vi "display_1s_stim_9s_ISI_CS1_CS2_no_trigger_with_probes.vi"() -> ()   [LabVIEW 2019]
uses:
  <vilib>/Analysis/Matrix/Datatypes/RealMatrix.ctl
  <vilib>/Utility/file.llb/Write Delimited Spreadsheet (DBL).vi
  <vilib>/Analysis/Matrix/NI_Matrix.lvlib
panel:
  out "Num trials":u32=204
  out "ISI Time":dbl
  out "Stim TS":dbl
  out "Output":dbl[][](array[numeric])
  out "Output frame":T1
  out "Array temp1":T1
  out "Elapsed Time":dbl
  out "Display":bool=TRUE
  out "Trial":u32=1
  out "reward":dbl[](array[numeric])
  out "stim_id":dbl[](array[numeric])
  out "stim_loaded":dbl
  out "Timings":dbl[](array[numeric])
  out "Stimuli Loaded?":bool
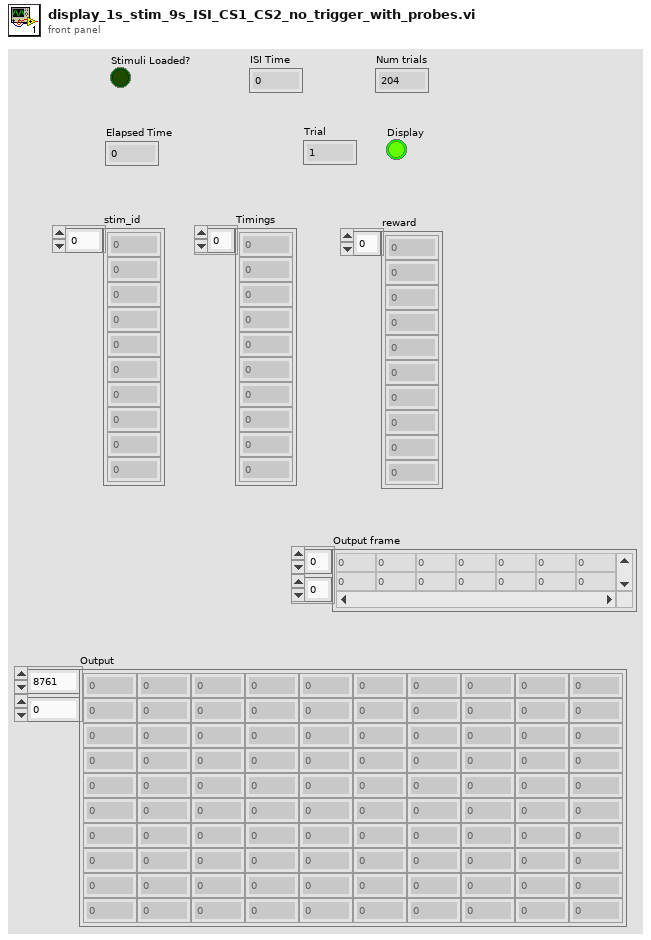
[diagram p1: front panel]
types:
  T1 = typedef "NI_Matrix.lvlib/RealMatrix.ctl" = dbl[][]
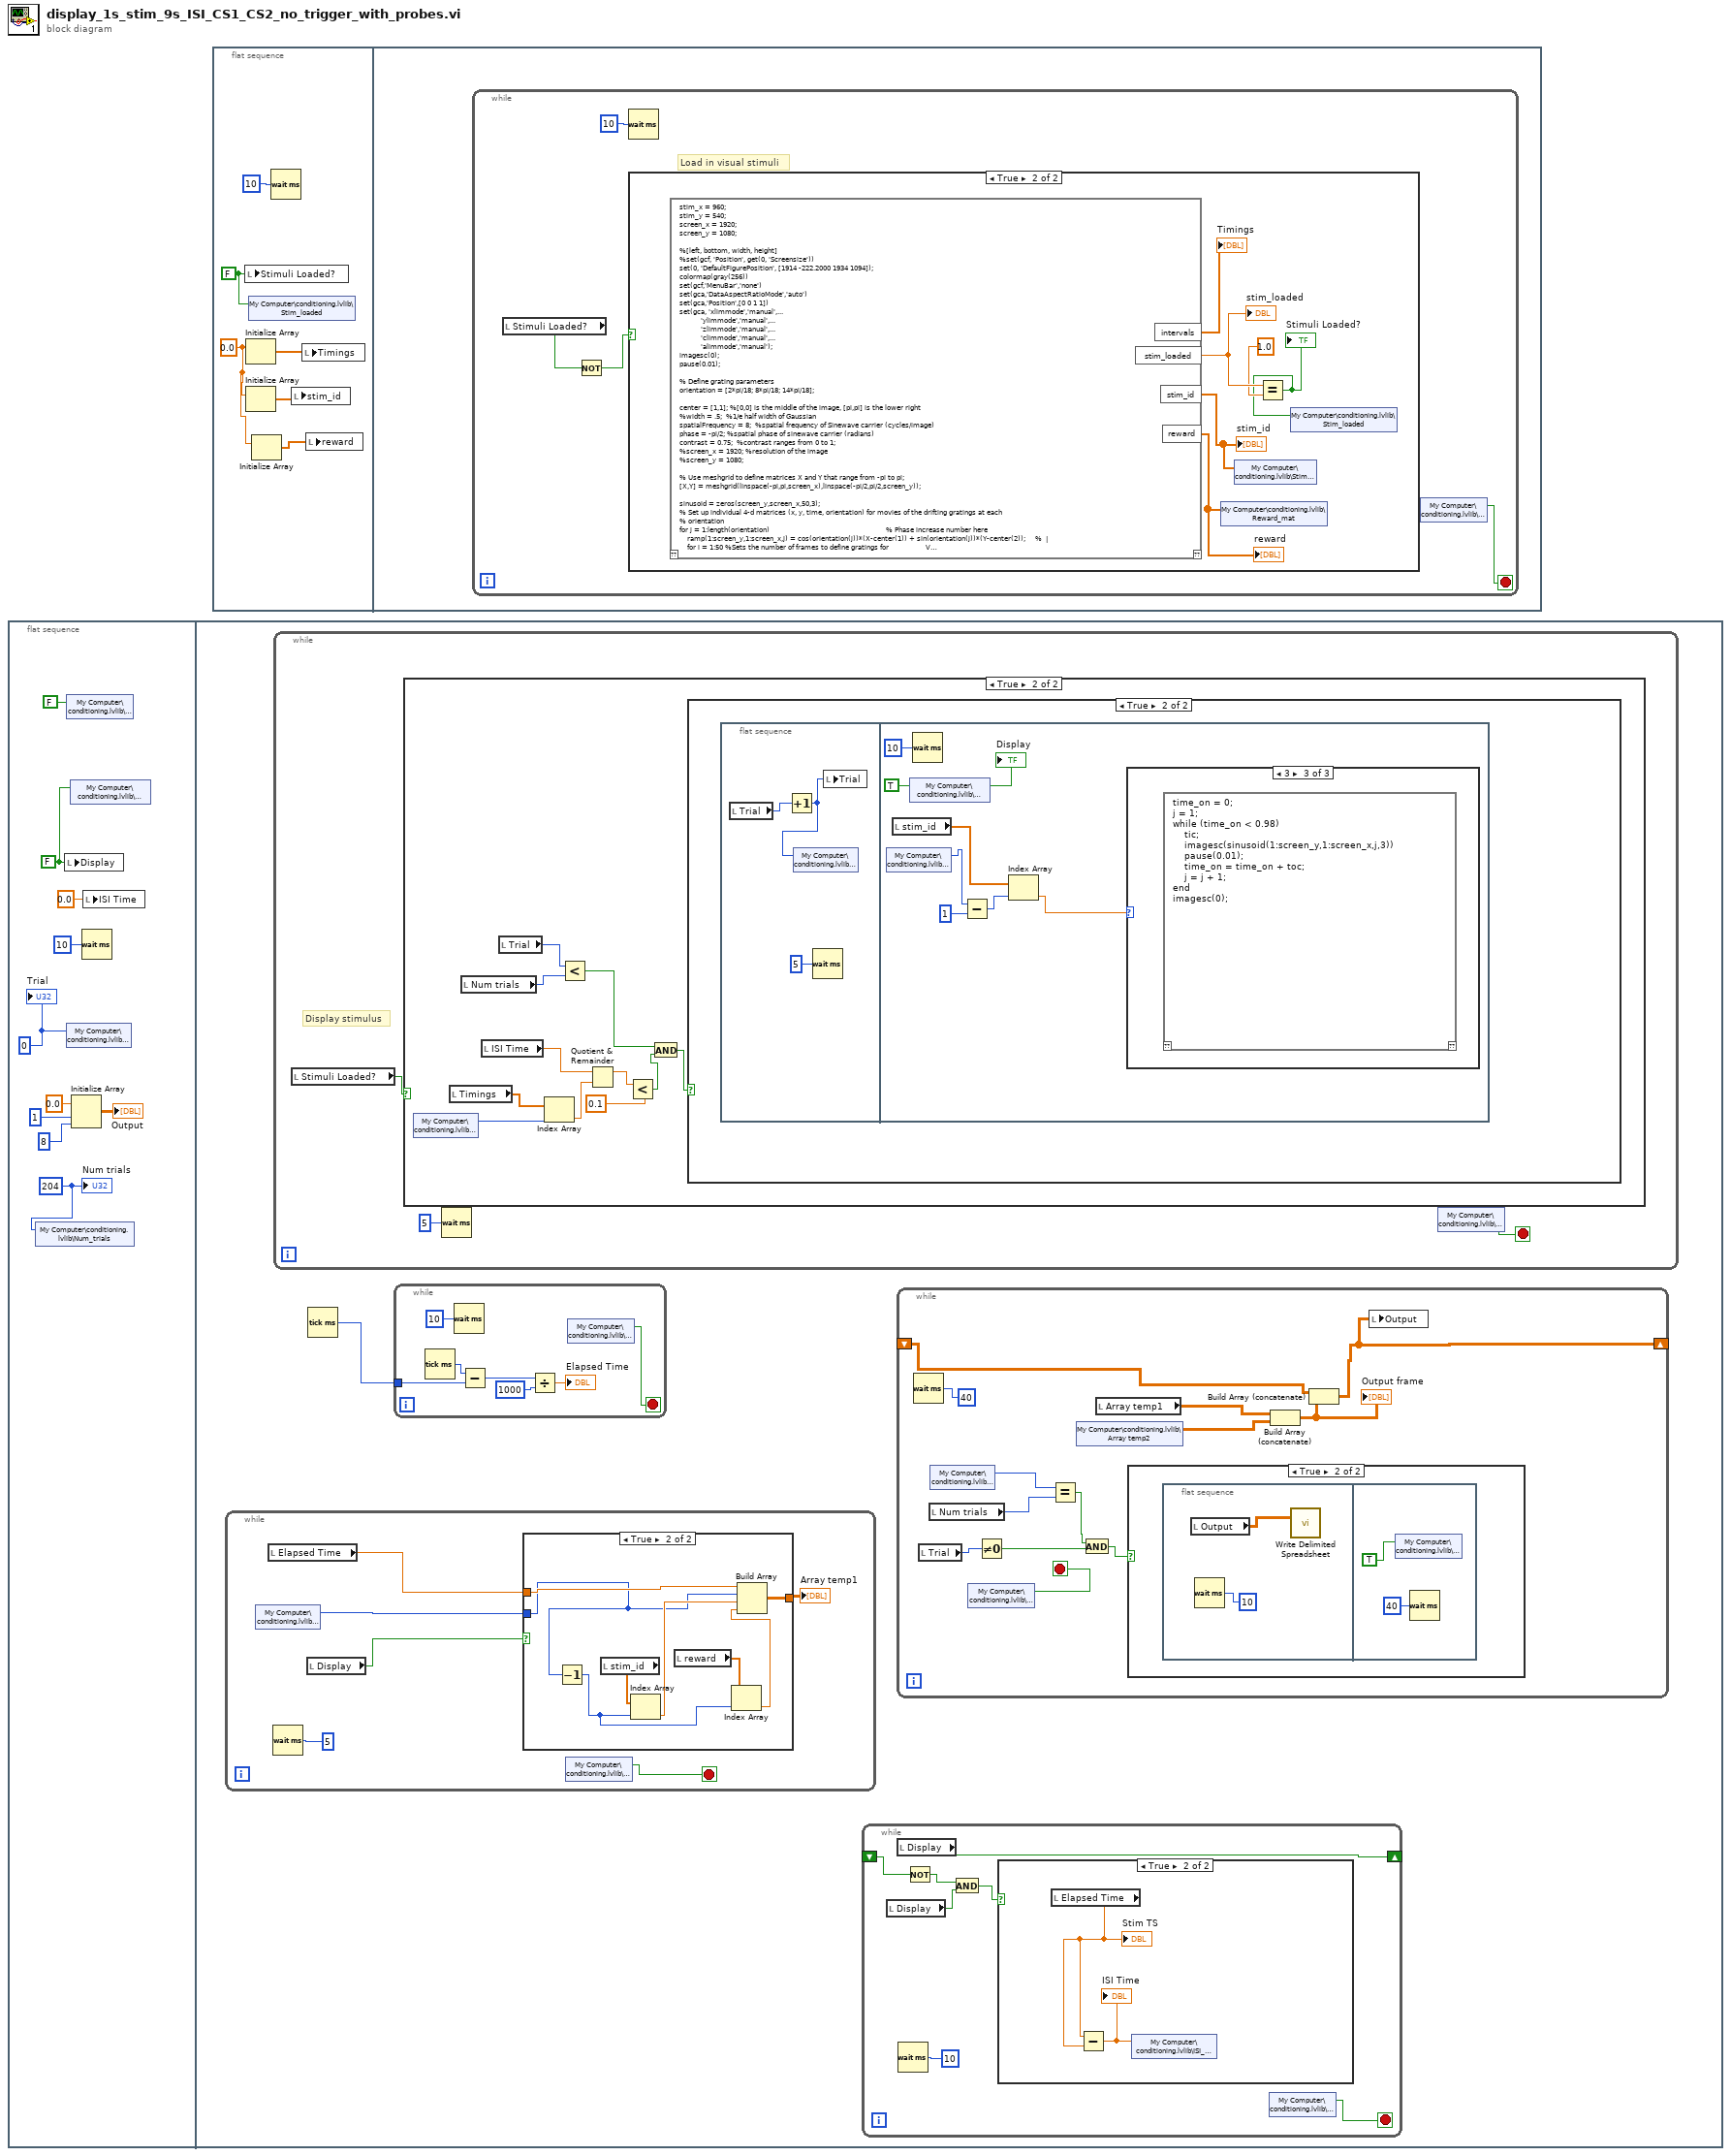
[diagram p0: block diagram]
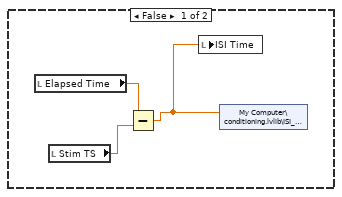
[diagram p3: hidden frame]
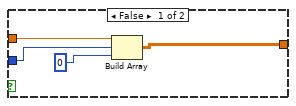
[diagram p4: hidden frame]
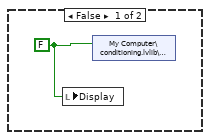
[diagram p7: hidden frame]
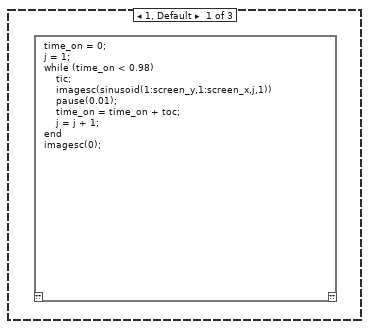
[diagram p8: hidden frame]
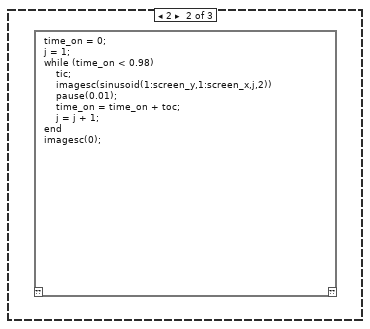
[diagram p9: hidden frame]
diagram:
  n1 = flat-sequence {
    frame #0 {
      w2 = u32 204
      w8 = FALSE ("Display")
      w10 = u32 0 ("Trial")
      n2 = shared-variable "My Computer\\conditioning.lvlib\\Num_trials"(w2) -> ()  [unwired: 1 in, 1 out]
      n3 = local write "Display"(w8) -> ()
      n4 = shared-variable "My Computer\\conditioning.lvlib\\Stop"(FALSE ("Stop")) -> ()  [unwired: 1 in, 1 out]
      n5 = shared-variable "My Computer\\conditioning.lvlib\\Trial"(w10) -> ()  [unwired: 1 in, 1 out]
      n6 = shared-variable "My Computer\\conditioning.lvlib\\Display"(w8) -> ()  [unwired: 1 in, 1 out]
      n7 = Initialize Array(0.0 ("element"), 1 ("dimension size"), 8 ("dimension size")) -> (→"Output":dbl[][])
      n8 = Wait (ms)(milliseconds to wait=u32 10) -> ()  [unwired: 1 out]
      n9 = local write "ISI Time"(0.0 ("ISI Time")) -> ()
      "Trial" <- w10
      "Num trials" <- w2
    }
    frame #1 {
      n10 = while {
        stop <- w24 stop-if-true
        n11 = shared-variable "My Computer\\conditioning.lvlib\\Trial"() -> (w26:u32)  [unwired: 1 in, 1 out]
        n12 = local read "Elapsed Time"() -> (w28:dbl)
        n13 = Wait (ms)(milliseconds to wait=u32 5) -> ()  [unwired: 1 out]
        n14 = local read "Display"() -> (w25:bool)
        n15 = case shown="True" w25 {
          tunnel: w26 -> [w32 w37]
          tunnel: w28 -> [w33 w39]
          tunnel: [w31 w40] -> w27
          frame False {
            n16 = Build Array(w33, w32, u32 0 ("milliseconds to wait")) -> (w31:T1)
          }
          frame True {
            n17 = Decrement(x=w37) -> (x-1=w35:u32)
            n18 = local read "stim_id"() -> (w41:dbl[])
            n19 = Index Array(array=w41, index=w35) -> (element=w38:dbl)
            n20 = local read "reward"() -> (w36:dbl[])
            n21 = Index Array(array=w36, index=w35) -> (element=w34:dbl)
            n22 = Build Array(w39, w37, w38, w34) -> (w40:T1)
          }
        }
        "Array temp1" <- w27
        n23 = shared-variable "My Computer\\conditioning.lvlib\\Stop"() -> (w24:bool)  [unwired: 1 in, 1 out]
      }
      n24 = while {
        stop <- w67 stop-if-true
        # "Display stimulus"
        n25 = local read "Stimuli Loaded?"() -> (w66:bool)
        n26 = case shown="True" w66 {
          frame False {
          }
          frame True {
            n27 = shared-variable "My Computer\\conditioning.lvlib\\Trial"() -> (w70:u32)  [unwired: 1 in, 1 out]
            n28 = local read "Timings"() -> (w77:dbl[])
            n29 = local read "Num trials"() -> (w69:u32)
            n30 = local read "ISI Time"() -> (w75:dbl)
            n31 = local read "Trial"() -> (w74:u32)
            n32 = Index Array(array=w77, index=w70) -> (element=w76:dbl)
            n33 = Less?(x=w74, y=w69) -> (x < y?=w73:bool)
            n34 = Quotient & Remainder(x=w75, y=w76) -> (x-y*floor(x/y)=w79:dbl)  [unwired: 1 out]
            n35 = Less?(x=w79, y=0.1) -> (x < y?=w72:bool)
            n36 = And(x=w73, y=w72) -> (x .and. y?=w71:bool)
            n37 = case shown="True" w71 {
              frame False {
                w80 = FALSE ("Display")
                n38 = local write "Display"(w80) -> ()
                n39 = shared-variable "My Computer\\conditioning.lvlib\\Display"(w80) -> ()  [unwired: 1 in, 1 out]
              }
              frame True {
                n40 = flat-sequence {
                  frame #0 {
                    n41 = local read "Trial"() -> (w82:u32)
                    n42 = Increment(x=w82) -> (x+1=w81:u32)
                    n43 = shared-variable "My Computer\\conditioning.lvlib\\Trial"(w81) -> ()  [unwired: 1 in, 1 out]
                    n44 = Wait (ms)(milliseconds to wait=u32 5) -> ()  [unwired: 1 out]
                    n45 = local write "Trial"(w81) -> ()
                  }
                  frame #1 {
                    w88 = TRUE ("Boolean")
                    n46 = shared-variable "My Computer\\conditioning.lvlib\\Trial"() -> (w86:u32)  [unwired: 1 in, 1 out]
                    n47 = local read "stim_id"() -> (w89:dbl[])
                    n48 = shared-variable "My Computer\\conditioning.lvlib\\Display"(w88) -> ()  [unwired: 1 in, 1 out]
                    n49 = Wait (ms)(milliseconds to wait=u32 10) -> ()  [unwired: 1 out]
                    n50 = Subtract(x=w86, y=u32 1) -> (x-y=w87:u32)
                    n51 = Index Array(array=w89, index=w87) -> (element=w84:dbl)
                    n52 = case shown="3" w84 {
                      frame 1, Default {
                        n53 = script code="time_on = 0;\nj = 1;\nwhile (time_on < 0.98)\n    tic;\n    imagesc(sinusoid(1:screen_y,1:screen_x,j,1))\n    pause(0.01);\n    time_on = time_on + toc;\n    j = j + 1;\nend\nimagesc(0);"() -> ()  [unwired: 1 in, 1 out]
                      }
                      frame 2 {
                        n54 = script code="time_on = 0;\nj = 1;\nwhile (time_on < 0.98)\n    tic;\n    imagesc(sinusoid(1:screen_y,1:screen_x,j,2))\n    pause(0.01);\n    time_on = time_on + toc;\n    j = j + 1;\nend\nimagesc(0);"() -> ()  [unwired: 1 in, 1 out]
                      }
                      frame 3 {
                        n55 = script code="time_on = 0;\nj = 1;\nwhile (time_on < 0.98)\n    tic;\n    imagesc(sinusoid(1:screen_y,1:screen_x,j,3))\n    pause(0.01);\n    time_on = time_on + toc;\n    j = j + 1;\nend\nimagesc(0);"() -> ()  [unwired: 1 in, 1 out]
                      }
                    }
                    "Display" <- w88
                  }
                }
              }
            }
          }
        }
        n56 = Wait (ms)(milliseconds to wait=u32 5) -> ()  [unwired: 1 out]
        n57 = shared-variable "My Computer\\conditioning.lvlib\\Stop"() -> (w67:bool)  [unwired: 1 in, 1 out]
      }
      n58 = Tick Count (ms)() -> (millisecond timer value=w11:u32)
      n59 = while {
        tunnel: w11 -> [w45]
        stop <- w42 stop-if-true
        n60 = Tick Count (ms)() -> (millisecond timer value=w46:u32)
        n61 = Wait (ms)(milliseconds to wait=u32 10) -> ()  [unwired: 1 out]
        n62 = Subtract(x=w46, y=w45) -> (x-y=w43:u32)
        n63 = Divide(x=w43, y=u32 1000) -> (x/y=→"Elapsed Time":dbl)
        n64 = shared-variable "My Computer\\conditioning.lvlib\\Stop"() -> (w42:bool)  [unwired: 1 in, 1 out]
      }
      n65 = while {
        shift-right: [w16] -> _
        shift-left: _ -> [w15]
        stop <- w18 stop-if-true
        n66 = local read "Display"() -> (w13:bool)
        n67 = local read "Display"() -> (w16:bool)
        n68 = Wait (ms)(milliseconds to wait=u32 10) -> ()  [unwired: 1 out]
        n69 = Not(x=w15) -> (.not. x?=w14:bool)
        n70 = And(x=w14, y=w13) -> (x .and. y?=w12:bool)
        n71 = case shown="True" w12 {
          frame False {
            n72 = local read "Elapsed Time"() -> (w19:dbl)
            n73 = local read "Stim TS"() -> (w21:dbl)
            n74 = Subtract(x=w19, y=w21) -> (x-y=w20:dbl)
            n75 = local write "ISI Time"(w20) -> ()
            n76 = shared-variable "My Computer\\conditioning.lvlib\\ISI_Time"(w20) -> ()  [unwired: 1 in, 1 out]
          }
          frame True {
            n77 = local read "Elapsed Time"() -> (w22:dbl)
            "Stim TS" <- w22
            n78 = Subtract(x=w22, y=w22) -> (x-y=w23:dbl)
            "ISI Time" <- w23
            n79 = shared-variable "My Computer\\conditioning.lvlib\\ISI_Time"(w23) -> ()  [unwired: 1 in, 1 out]
          }
        }
        n80 = shared-variable "My Computer\\conditioning.lvlib\\Stop"() -> (w18:bool)  [unwired: 1 in, 1 out]
      }
      n81 = while {
        shift-right: [w58] -> _
        shift-left: _ -> [w59]
        stop <- w61 stop-if-true
        n82 = Wait (ms)(milliseconds to wait=u32 40) -> ()  [unwired: 1 out]
        n83 = local read "Trial"() -> (w51:u32)
        n84 = local read "Num trials"() -> (w53:u32)
        n85 = shared-variable "My Computer\\conditioning.lvlib\\Trial"() -> (w54:u32)  [unwired: 1 in, 1 out]
        n86 = shared-variable "My Computer\\conditioning.lvlib\\Stop"() -> (w61:bool)  [unwired: 1 in, 1 out]
        n87 = Not Equal To 0?(x=w51) -> (x != 0?=w50:bool)
        n88 = Equal?(x=w54, y=w53) -> (x = y?=w52:bool)
        n89 = shared-variable "My Computer\\conditioning.lvlib\\Array temp2"() -> (w56:dbl[][])  [unwired: 1 in, 1 out]
        n90 = And(x=w52, y=w50) -> (x .and. y?=w49:bool)
        n91 = local read "Array temp1"() -> (w57:T1)
        n92 = case shown="True" w49 {
          frame False {
          }
          frame True {
            n93 = flat-sequence {
              frame #0 {
                n94 = local read "Output"() -> (w63:dbl[][])
                n95 = Wait (ms)(milliseconds to wait=u32 10) -> ()  [unwired: 1 out]
                n96 = call-poly <vilib>:"Write Delimited Spreadsheet.vi"("2D data"=w63) -> ()  [unwired: 13 in, 2 out]
              }
              frame #1 {
                n97 = shared-variable "My Computer\\conditioning.lvlib\\Stop"(TRUE) -> ()  [unwired: 1 in, 1 out]
                n98 = Wait (ms)(milliseconds to wait=u32 40) -> ()  [unwired: 1 out]
              }
            }
          }
        }
        n99 = Build Array (concatenate)(w57, w56) -> (w55:T1)
        "Output frame" <- w55
        n100 = Build Array (concatenate) ("Build Matrix")(w59, w55) -> (w58:T1)
        n101 = local write "Output"(w58) -> ()
      }
    }
  }
  n102 = flat-sequence {
    frame #0 {
      w93 = 0.0 ("element")
      w91 = FALSE ("Stimuli Loaded?")
      n103 = local write "Stimuli Loaded?"(w91) -> ()
      n104 = Initialize Array(w93) -> (w95:dbl[])  [unwired: 1 in]
      n105 = Initialize Array(w93) -> (w94:dbl[])  [unwired: 1 in]
      n106 = shared-variable "My Computer\\conditioning.lvlib\\Stim_loaded"(w91) -> ()  [unwired: 1 in, 1 out]
      n107 = Initialize Array(w93) -> (w92:dbl[])  [unwired: 1 in]
      n108 = Wait (ms)(milliseconds to wait=u32 10) -> ()  [unwired: 1 out]
      n109 = local write "stim_id"(w94) -> ()
      n110 = local write "Timings"(w95) -> ()
      n111 = local write "reward"(w92) -> ()
    }
    frame #1 {
      n112 = while {
        stop <- w99 stop-if-true
        # "Load in visual stimuli"
        n113 = local read "Stimuli Loaded?"() -> (w98:bool)
        n114 = Not(x=w98) -> (.not. x?=w97:bool)
        n115 = Wait (ms)(milliseconds to wait=u32 10) -> ()  [unwired: 1 out]
        n116 = case shown="True" w97 {
          frame False {
          }
          frame True {
            n117 = script code="stim_x = 960;\nstim_y = 540;\nscreen_x = 1920;\nscreen_y = 1080;\n\n%[left, bottom, width, height]\n%set(gcf, 'Position', get(0, 'Screensize'))\nset(0, 'DefaultFigurePosition', [1914 -222.2000 1934 1094]);\ncolormap(gray(256))\nset(gcf,'MenuBar','none')\nset(gca,'DataAspectRatioMode','auto')\nset(gca,'Position',[0 0 1 1])\nset(gca, 'xlimmode','manual',...\n           'ylimmode','manual',...\n           'zlimmode','manual',...\n           'climmode','manual',...\n           'alimmode','manual');\nimagesc(0);\npause(0.01);\n\n% Define grating parameters\norientation = [2*pi/18; 8*pi/18; 14*pi/18];\n\ncenter = [1,1]; %[0,0] is the middle of the image, [pi,pi] is the lower right\n%width = .5;  %1/e half width of Gaussian\nspatialFrequency = 8;  %spatial frequency of Sinewave carrier (cycles/image)\nphase = -pi/2; %spatial phase of sinewave carrier (radians)\ncontrast = 0.75;  %contrast ranges from 0 to 1;\n%screen_x = 1920; %resolution of the image  \n%screen_y = 1080;\n\n% Use meshgrid to define matrices X and Y that range from -pi to pi;\n[X,Y] = meshgrid(linspace(-pi,pi,screen_x),linspace(-pi/2,pi/2,screen_y));\n\nsinusoid = zeros(screen_y,screen_x,50,3);\n% Set up individual 4-d matrices (x, y, time, orientation) for movies of the drifting gratings at each\n% orientation\nfor j = 1:length(orientation)                                                            % Phase increase number here\n    ramp(1:screen_y,1:screen_x,j) = cos(orientation(j))*(X-center(1)) + sin(orientation(j))*(Y-center(2));     %  |\n    for i = 1:50 %Sets the number of frames to define gratings for                   V\n       sinusoid(1:screen_y,1:screen_x,i,j) = contrast*sin(spatialFrequency*ramp(1:screen_y,1:screen_x,j)-...\n           (phase+(2*pi*(i-1)*(-30)/360))); %Number before '/360' sets the phase increase\n    end\nend\n\nintervals = [ones(1,41)*10 ones(1,41)*11 ones(1,41)*12 ones(1,41)*13 ones(1,40)*14];\nintervals = intervals(randperm(204));\nrand_idx1 = randperm(204);\nrand_idx2 = randperm(204);\nstim_id = [ones(1,102)*1 ones(1,102)*2];\nreward = [ones(1,87)*1 ones(1,15)*0 ones(1,87)*1 ones(1,15)*0];\nstim_id = stim_id(rand_idx2);\nreward = reward(rand_idx2);\n\nstim_loaded = 1;" ("Script Node")() -> ("stim_loaded"=w106:dbl, "intervals"=→"Timings":dbl[], "stim_id"=w101:dbl[], "reward"=w103:dbl[])  [unwired: 1 in, 1 out]
            "stim_loaded" <- w106
            "stim_id" <- w101
            "reward" <- w103
            n118 = shared-variable "My Computer\\conditioning.lvlib\\Reward_mat"(w103) -> ()  [unwired: 1 in, 1 out]
            n119 = shared-variable "My Computer\\conditioning.lvlib\\Stim_ID"(w101) -> ()  [unwired: 1 in, 1 out]
            n120 = Equal?(x=w106, y=1.0) -> (x = y?=w102:bool)
            "Stimuli Loaded?" <- w102
            n121 = shared-variable "My Computer\\conditioning.lvlib\\Stim_loaded"(w102) -> ()  [unwired: 1 in, 1 out]
          }
        }
        n122 = shared-variable "My Computer\\conditioning.lvlib\\Stop"() -> (w99:bool)  [unwired: 1 in, 1 out]
      }
    }
  }
